vi "Database Path.vi"(8 "error in (no error)":errorcluster, 10 "Database path":path, 11 "Paquetes Disponibles in":refnum<class "Paquetes Disponibles.lvclass">) -> (0 "error out":errorcluster, 3 "Paquetes Disponibles out":refnum<class "Paquetes Disponibles.lvclass">)   [LabVIEW 2020, in "Paquetes Disponibles.lvlib" / "Paquetes Disponibles.lvclass"]
uses:
  Paquetes Disponibles.lvclass
  Paquetes Disponibles.lvclass/Paquetes Disponibles.ctl
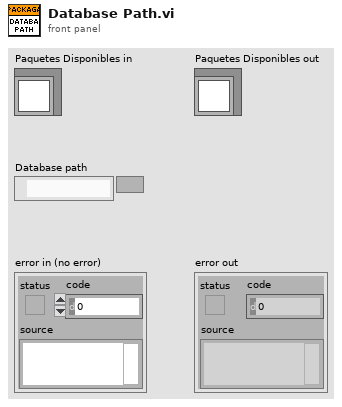
[diagram p1: front panel]
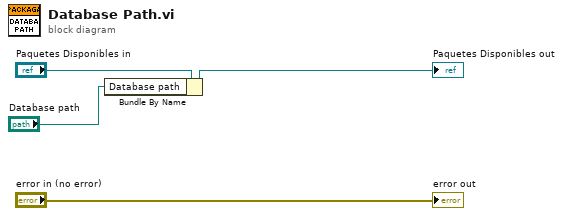
[diagram p0: block diagram]
diagram:
  n1 = Bundle By Name(cluster="Paquetes Disponibles in", "Database path"="Database path") -> (→"Paquetes Disponibles out":refnum<class "Paquetes Disponibles.lvclass">)
  "error out" <- "error in (no error)"
